vi "CSC_SetLegLength.vi"(8 "error in (no error)":errorcluster, 10 "LegLength":T1={"Thigh Length (m)"=0.446, "Shank Length (m)"=0.446}, 11 "C-Alex in":refnum<class "CableSerialChain.lvclass">) -> (0 "error out":errorcluster, 3 "C-Alex out":refnum<class "CableSerialChain.lvclass">)   [LabVIEW 2014]
uses:
  Body/Bodies.lvclass
  Body/PointOnBody.ctl
  CableSerialChain.lvclass
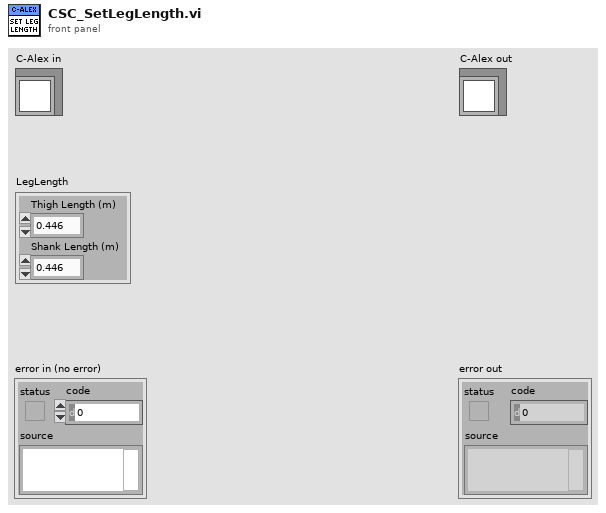
[diagram p1: front panel]
types:
  T1 = cluster{"Thigh Length (m)":dbl, "Shank Length (m)":dbl}
  T2 = typedef "Bodies.lvclass/PointOnBody.ctl" = cluster{"Coord4":dbl[], "ID":i32}
  T3 = cluster{"DH":cluster{enum16{"Theta", "Alpha", "a", "d"}, dbl}[], "CoM_Pos":T2, "Mass(kg)":dbl}
  T4 = cluster{enum16{"Theta", "Alpha", "a", "d"}, dbl}[]
  T5 = cluster{"DH":cluster{enum16{"Theta", "Alpha", "a", "d"}, dbl}[], "CoM_Pos":T2, "Mass(kg)":dbl}[]
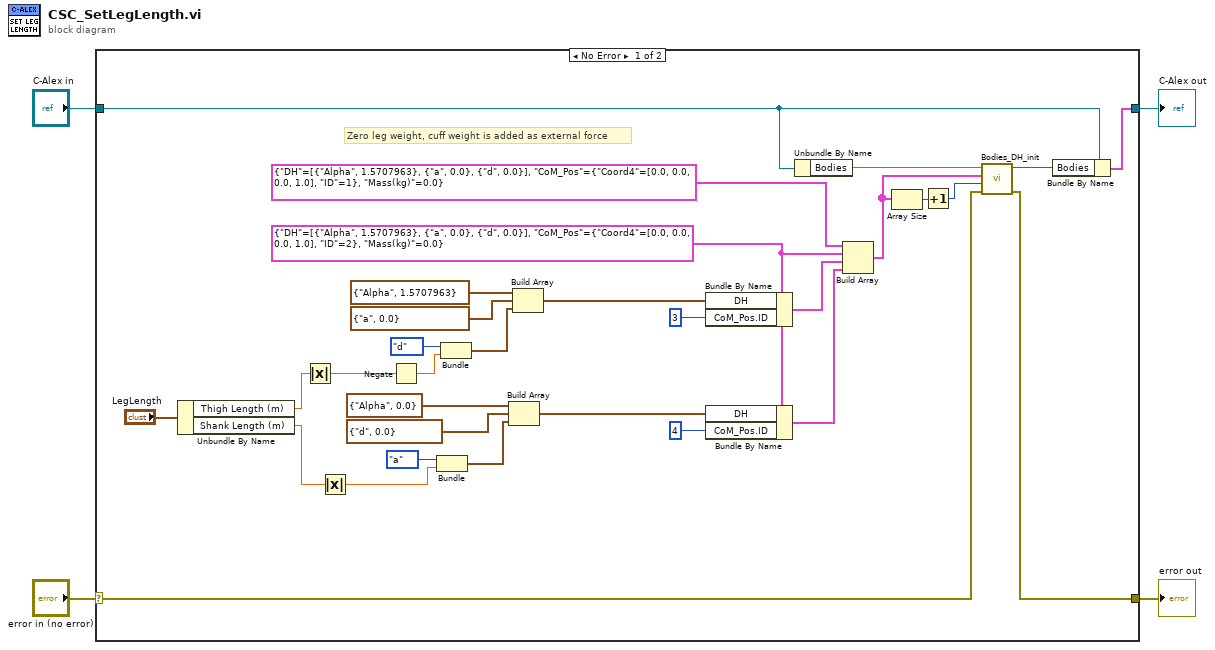
[diagram p0: block diagram]
diagram:
  n1 = case shown="No Error" "error in (no error)" {
    selector: "error in (no error)" -> [w30 w37]
    tunnel: [w31 w37] -> w3
    tunnel: [w34 w36] -> w1
    tunnel: "C-Alex in" -> [w35 w36]
    frame No Error {
      w12 = T3 {"DH"=[{enum."Alpha", 1.5707963}, {enum."a", 0.0}, {enum."d", 0.0}], "CoM_Pos"={"Coord4"=[0.0, 0.0, 0.0, 1.0], "ID"=2}, "Mass(kg)"=0.0}
      # "Zero leg weight, cuff weight is added as external force"
      n2 = Unbundle By Name("LegLength") -> ("Thigh Length (m)"=w8:dbl, "Shank Length (m)"=w7:dbl)
      n3 = Absolute Value(x=w8) -> (abs(x)=w6:dbl)
      n4 = Absolute Value(x=w7) -> (abs(x)=w5:dbl)
      n5 = Negate(x=w6) -> (-x=w26:dbl)
      n6 = Bundle(enum16{"Theta", "Alpha", "a", "d"}."a", w5) -> (w20:cluster{enum16{"Theta", "Alpha", "a", "d"}, dbl})  [unwired: 1 in]
      n7 = Bundle(enum16{"Theta", "Alpha", "a", "d"}."d", w26) -> (w25:cluster{enum16{"Theta", "Alpha", "a", "d"}, dbl})  [unwired: 1 in]
      n8 = Build Array(cluster{enum16{"Theta", "Alpha", "a", "d"}, dbl} {enum."Alpha", 0.0}, cluster{enum16{"Theta", "Alpha", "a", "d"}, dbl} {enum."d", 0.0}, w20) -> (w15:T4)
      n9 = Build Array(cluster{enum16{"Theta", "Alpha", "a", "d"}, dbl} {enum."Alpha", 1.5707963}, cluster{enum16{"Theta", "Alpha", "a", "d"}, dbl} {enum."a", 0.0}, w25) -> (w18:T4)
      n10 = Bundle By Name(cluster=w12, "DH"=w18, "CoM_Pos.ID"=3 ("CoM_Pos.Body ID")) -> (w13:T3)
      n11 = Bundle By Name(cluster=w12, "DH"=w15, "CoM_Pos.ID"=4 ("CoM_Pos.Body ID")) -> (w14:T3)
      n12 = Unbundle By Name(w35) -> ("Bodies"=w32)
      n13 = Build Array(T3 {"DH"=[{enum."Alpha", 1.5707963}, {enum."a", 0.0}, {enum."d", 0.0}], "CoM_Pos"={"Coord4"=[0.0, 0.0, 0.0, 1.0], "ID"=1}, "Mass(kg)"=0.0}, w12, w13, w14) -> (w10:T5)
      n14 = Array Size(array=w10) -> (size(s)=w29:i32)
      n15 = Increment(x=w29) -> (x+1=w28:i32)
      n16 = call "Bodies_DH_init.vi"("error in (no error)"=w30, "Number of Bodies (Including Base)"=w28, "KnownDHVars"=w10, "Body.lvclass In"=w32) -> ("error out"=w31:errorcluster, "Body.lvclass Out"=w33:refnum<class "Bodies.lvclass">)  [unwired: 6 in]
      n17 = Bundle By Name(cluster=w35, "Bodies"=w33) -> (w34:cluster{})
    }
    frame Error {
    }
  }
  "error out" <- w3
  "C-Alex out" <- w1
